vi "Chart UI Module.vi"() -> ()   [LabVIEW 2014]
uses:
  Communication/Events/Events Lib.lvlib
panel:
  out "error out":errorcluster
  in  "Stop":bool
  out "Chart":dbl(graph)
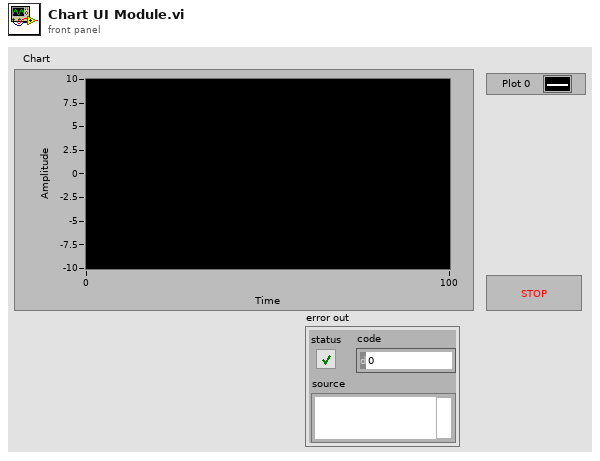
[diagram p1: front panel]
types:
  T1 = typedef "Events Lib.lvlib/Events TypeDef.ctl" = cluster{"Stop Event":refnum<user-event>, "Chart Send Value":refnum<user-event>}
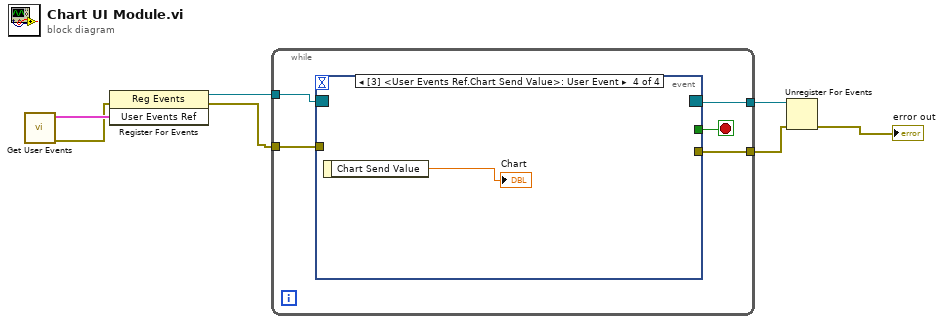
[diagram p0: block diagram]
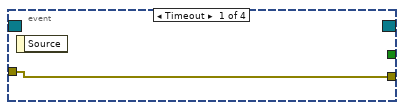
[diagram p2: hidden frame]
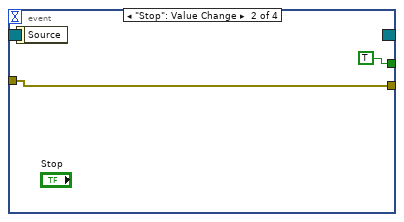
[diagram p3: hidden frame]
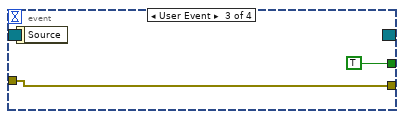
[diagram p4: hidden frame]
diagram:
  n1 = call "Get User Events.vi"() -> ("error out"=w5:errorcluster, "User Events Ref"=w6:T1)  [unwired: 10 in]
  n2 = register-events(error in=w5, w6) -> (reference out=w7:refnum<event-registration>, error out=w4:errorcluster)  [unwired: 1 in]
  n3 = while {
    tunnel: w7 -> [w12]
    tunnel: w4 -> [w11]
    tunnel: [w9] -> w3
    tunnel: [w8] -> w2
    stop <- w10 stop-if-true
    n4 = event shown="[3] <User Events Ref.Chart Send Value>: User Event" {
      selector: w12 -> [_ _ _ _]
      dyn-events: [_ _ _ _] -> w9
      timeout: _ -> [_ _ _ _]
      tunnel: w11 -> [w13 w14 w16 _]
      tunnel: [_ TRUE TRUE _] -> w10
      tunnel: [w13 w14 w16 _] -> w8
      event Timeout {
        n5 = event-data() -> ()  [unwired: 1 in, 1 out]
      }
      event "Stop": Value Change {
        n6 = event-data() -> ()  [unwired: 1 in, 1 out]
      }
      event User Event {
        n7 = event-data() -> ()  [unwired: 1 in, 1 out]
      }
      event User Event {
        n8 = event-data() -> ("Chart Send Value"=→"Chart":dbl)  [unwired: 1 in]
      }
    }
  }
  n9 = Unregister For Events(event registration refnum=w3, error in=w2) -> (error out=→"error out":errorcluster)
